vi "Process Coin.vi"(8 "error in (no error)":errorcluster, 10 "Coins":cluster{"1":bool, "2":bool, "5":bool}, 11 "MXN Actor in":refnum<class "MXN Actor.lvclass">) -> (0 "error out":errorcluster, 3 "MXN Actor out":refnum<class "MXN Actor.lvclass">)   [LabVIEW 2020, in "MXN Actor.lvlib" / "MXN Actor.lvclass"]
uses:
  MXN Actor.lvclass
  C:/Program Files/National Instruments/LabVIEW 2020/vi.lib/ActorFramework/Actor/Actor.lvclass
  <vilib>/ActorFramework/Actor/Actor.lvclass/Actor.ctl
  MXN Actor.lvclass/MXN Actor.ctl
  UI Actor Messages/Credit Update Msg/Credit Update Msg.lvclass/Credit Update Msg.ctl
  <vilib>/ActorFramework/Message Enqueuer/Message Enqueuer.lvclass/Message Enqueuer.ctl
  <vilib>/ActorFramework/Message Enqueuer/Enqueue.vi
  UI Actor Messages/Credit Update Msg/Credit Update Msg.lvclass
  C:/Program Files/National Instruments/LabVIEW 2020/vi.lib/ActorFramework/Message/Message.lvclass
  <vilib>/ActorFramework/Message Priority Queue/Priority Enqueue.vi
  <vilib>/ActorFramework/Actor/Actor.lvclass
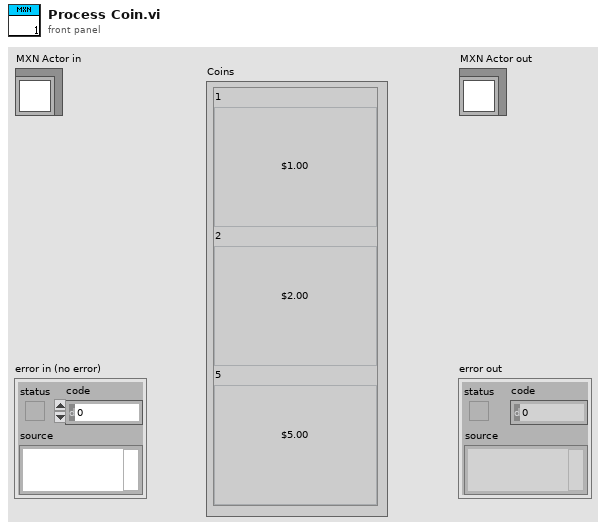
[diagram p1: front panel]
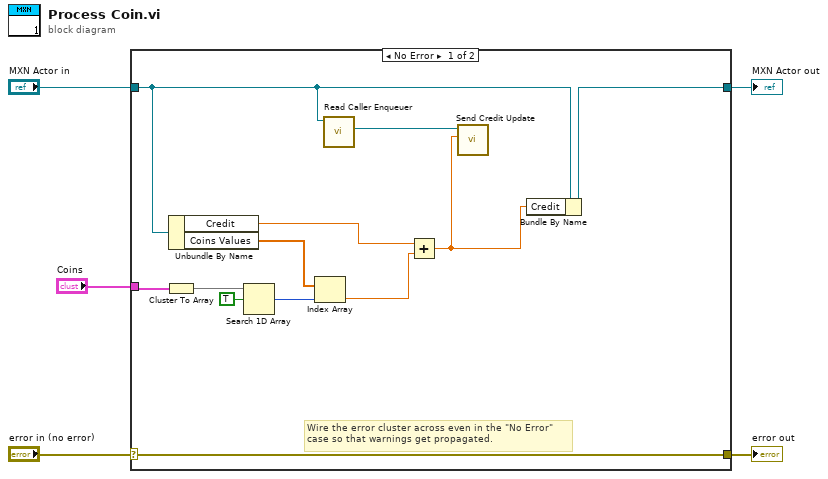
[diagram p0: block diagram]
diagram:
  n1 = case shown="No Error" "error in (no error)" {
    selector: "error in (no error)" -> [w17 w19]
    tunnel: [w17 w19] -> w4
    tunnel: [w9 w18] -> w2
    tunnel: "MXN Actor in" -> [w8 w18]
    tunnel: "Coins" -> [w16 _]
    frame No Error {
      # "Wire the error cluster across even in the \"No Error\"\ncase so that warnings get propagated."
      n2 = Cluster To Array(cluster=w16) -> (array=w15:bool[])
      n3 = Unbundle By Name(w8) -> ("Credit"=w10:dbl, "Coins Values"=w13:dbl[])
      n4 = Search 1D Array(1D array=w15, element=TRUE) -> (index of element=w12:i32)  [unwired: 1 in]
      n5 = Index Array(array=w13, index=w12) -> (element=w11:dbl)
      n6 = call <vilib>:"Read Caller Enqueuer.vi"("Actor"=w8) -> ("Caller Enqueuer"=w7:refnum<class "Message Enqueuer.lvclass">)  [unwired: 10 in]
      n7 = Add(x=w10, y=w11) -> (x+y=w6:dbl)
      n8 = call "Send Credit Update.vi"("Credit"=w6, "Message Enqueuer"=w7) -> ()  [unwired: 8 in, 2 out]
      n9 = Bundle By Name(cluster=w8, "Credit"=w6) -> (w9:refnum<class "MXN Actor.lvclass">)
    }
    frame Error {
    }
  }
  "error out" <- w4
  "MXN Actor out" <- w2
